vi "GetClassLocation.vi"(8 "ErrorIn":errorcluster, 10 "ClassString":string) -> (0 "ErrorOut":errorcluster, 2 "ClassFilePath":path)   [LabVIEW 2021, in "Application.lvclass"]
uses:
  Application.lvclass
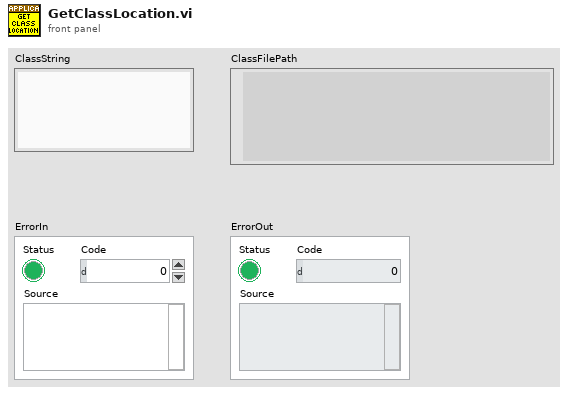
[diagram p1: front panel]
types:
  T1 = typedef "Application.lvclass/ObjectAttributes.ctl" = cluster{"Objects":variant, "BasePath":path, "Application":refnum<class "Application.lvclass">}
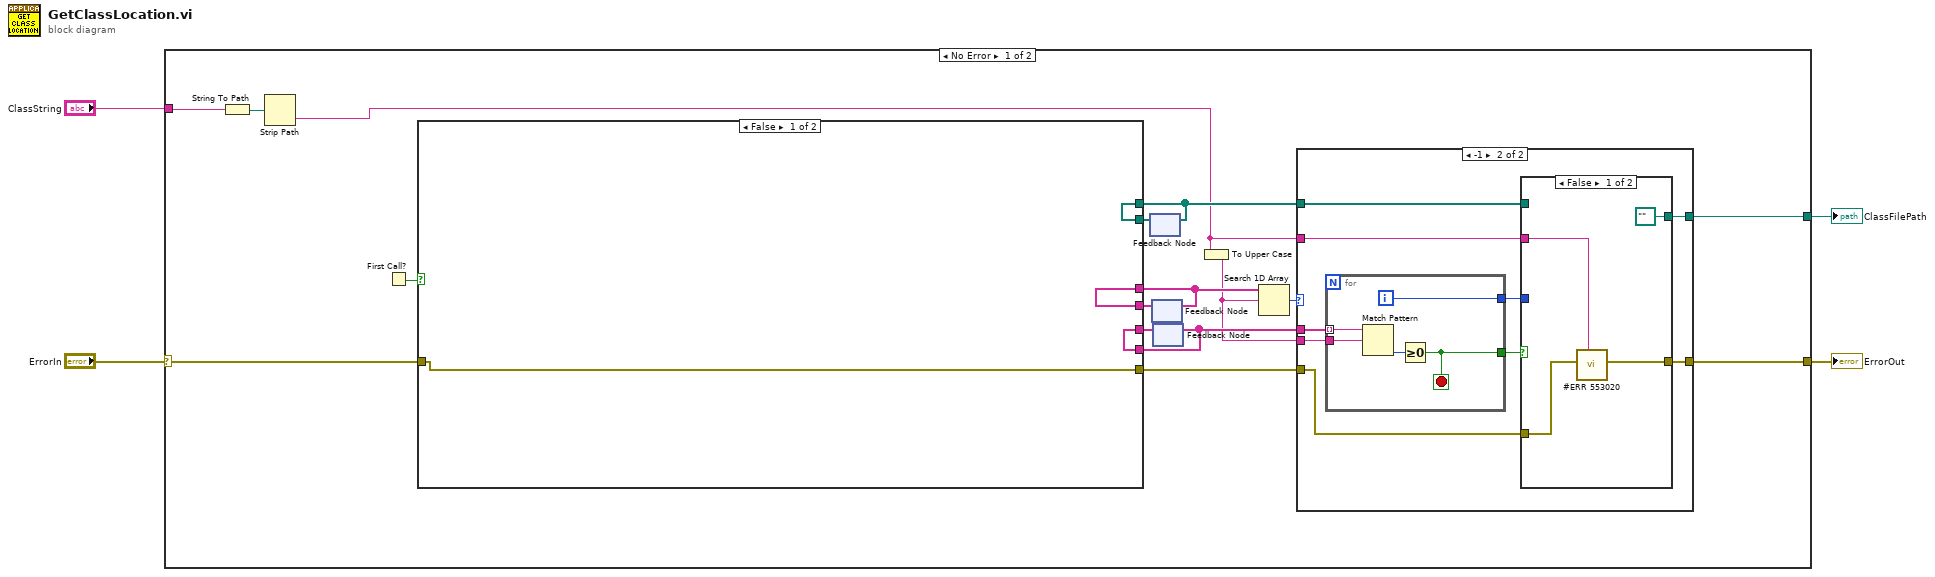
[diagram p0: block diagram]
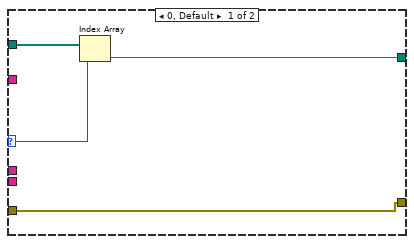
[diagram p2: hidden frame]
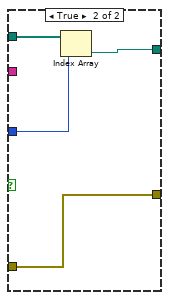
[diagram p3: hidden frame]
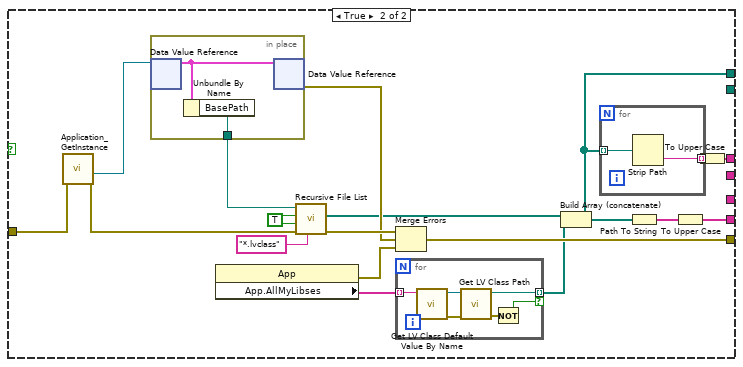
[diagram p4: hidden frame]
diagram:
  n1 = case shown="No Error" "ErrorIn" {
    selector: "ErrorIn" -> [w20 w79]
    tunnel: [w18 w79] -> w3
    tunnel: "ClassString" -> [w7 _]
    tunnel: [w10 _] -> w1
    frame No Error {
      n2 = String To Path(string=w7) -> (path=w6:path)
      n3 = Strip Path(path=w6) -> (name=w5:string)  [unwired: 1 out]
      n4 = First Call?() -> (First Call?: T/F=w17:bool)
      n5 = feedback #1() -> (w8:path[])  [unwired: 1 in]
      n6 = feedback #2() -> (w16:string[])  [unwired: 1 in]
      n7 = feedback #3() -> (w15:string[])  [unwired: 1 in]
      n8 = case shown="False" w17 {
        tunnel: w20 -> [w50 w68]
        tunnel: [w50 w65] -> w19
        tunnel: [w48 w51] -> w12
        tunnel: [w49 w52] -> w14
        tunnel: w16 -> [w49 _]
        tunnel: w15 -> [w48 _]
        tunnel: [w47 w53] -> w9
        tunnel: w8 -> [w47 _]
        frame False {
        }
        frame True {
          w60 = TRUE ("Treat LLBs as Folders?")
          n9 = call "Application_GetInstance.vi"("ErrorIn"=w68) -> ("ErrorOut"=w66:errorcluster, "DVRRefOut"=w62:refnum<data-value>)  [unwired: 6 in, 3 out]
          n10 = in-place {
            in-place-border: [w77] -> w59
            n11 = in-place-dvr #4(w62) -> (w78:T1)  [unwired: 1 out]
            n12 = Unbundle By Name(w78) -> ("BasePath"=w77:path)
            n13 = in-place-dvr #4(w78) -> (w64:errorcluster)  [unwired: 1 out]
          }
          n14 = property class="App"() -> (error out=w63:errorcluster, "App.AllMyLibses"=w58:string[])  [unwired: 2 in, 1 out]
          n15 = call <vilib>:"Recursive File List.vi"("pattern"="*.lvclass", "error in (no error)"=w66, "Continue Recursing on Error? (F)"=w60, "Treat LLBs as Folders?"=w60, "Folder Path"=w59) -> ("error out"=w67:errorcluster, "All Files in Dir"=w57:path[])  [unwired: 2 in, 3 out]
          n16 = Merge Errors(w67, w64, w63) -> (w65:errorcluster)
          n17 = for {
            tunnel: w58 -> [w74] mode=indexing
            tunnel: [w72] -> w56 mode=indexing if=w71
            n18 = call <vilib>:"Get LV Class Default Value By Name.vi"("class name"=w74) -> ("error out"=w76:errorcluster, "object"=w73:refnum<class>)  [unwired: 9 in]
            n19 = call <vilib>:"Get LV Class Path.vi"("error in (no error)"=w76, "object"=w73) -> ("error out"=w75:errorcluster, "class path"=w72:path)  [unwired: 8 in]
            n20 = Not(x=w75) -> (.not. x?=w71:bool)
          }
          n21 = Build Array (concatenate)(w57, w56) -> (w53:path[])
          n22 = for {
            tunnel: w53 -> [w70] mode=indexing
            tunnel: [w69] -> w54 mode=indexing
            n23 = Strip Path(path=w70) -> (name=w69:string)  [unwired: 1 out]
          }
          n24 = Path To String(path=w53) -> (string=w55:string[])
          n25 = To Upper Case(1:w55) -> (0:w51:string[])
          n26 = To Upper Case(1:w54) -> (0:w52:string[])
        }
      }
      n27 = feedback-in #1(w9) -> ()
      n28 = feedback-in #2(w14) -> ()
      n29 = feedback-in #3(w12) -> ()
      n30 = To Upper Case(1:w5) -> (0:w11:string)
      n31 = Search 1D Array(1D array=w14, element=w11) -> (index of element=w13:i32)  [unwired: 1 in]
      n32 = case shown="-1" w13 {
        selector: w13 -> [w22 _]
        tunnel: w12 -> [_ w31]
        tunnel: w11 -> [_ w30]
        tunnel: w9 -> [w23 w28]
        tunnel: [w21 w26] -> w10
        tunnel: w19 -> [w24 w32]
        tunnel: [w24 w33] -> w18
        tunnel: w5 -> [_ w25]
        frame 0, Default {
          n33 = Index Array(array=w23, index=w22) -> (element=w21:path)
        }
        frame -1 {
          n34 = for {
            tunnel: w31 -> [w46] mode=indexing
            tunnel: w30 -> [w45]
            tunnel: [w43] -> w27
            tunnel: [w42] -> w29
            i -> [w43]
            stop <- w42 stop-if-true
            n35 = Match Pattern(string=w46, regular expression=w45) -> (offset past match=w44:i32)  [unwired: 1 in, 3 out]
            n36 = Greater Or Equal To 0?(x=w44) -> (x >= 0?=w42:bool)
          }
          n37 = case shown="False" w29 {
            tunnel: w28 -> [_ w40]
            tunnel: w27 -> [_ w39]
            tunnel: [path "" ("class path") w38] -> w26
            tunnel: [w37 w41] -> w33
            tunnel: w32 -> [w36 w41]
            tunnel: w25 -> [w34 _]
            frame False {
              n38 = call "#ERR 553020"("Data"=w34, "error in (no error)"=w36) -> ("error out"=w37:errorcluster)  [unwired: 9 in]
            }
            frame True {
              n39 = Index Array(array=w40, index=w39) -> (element=w38:path)
            }
          }
        }
      }
    }
    frame Error {
    }
  }
  "ErrorOut" <- w3
  "ClassFilePath" <- w1
